vi "Get or Create Virtual Instrument.vi"(8 "Error In":errorcluster, 10 "Virtual Instrument Identifier":string) -> (0 "Error Out":errorcluster, 2 "IVritual Instrument":refnum<class "IVirtual Instrument.lvclass">)   [LabVIEW 2024, in "Instrument Manager.lvclass"]
uses:
  Instrument Manager.lvclass
  Interfaces/IVirtual Instrument/IVirtual Instrument.lvclass
  Instrument Manager.lvclass/Instrument Manager.ctl
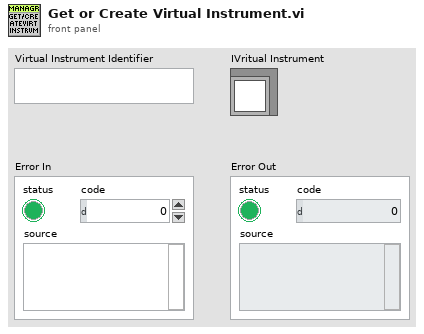
[diagram p1: front panel]
types:
  T1 = map{string, refnum<class "IVirtual Instrument.lvclass">}
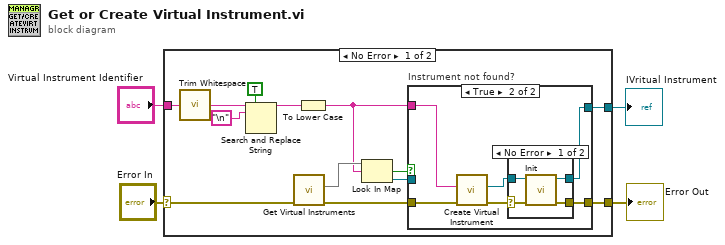
[diagram p0: block diagram]
diagram:
  n1 = case shown="No Error" "Error In" {
    selector: "Error In" -> [w5 w32]
    tunnel: [w17 w32] -> w4
    tunnel: [w12 _] -> w3
    tunnel: "Virtual Instrument Identifier" -> [w11 _]
    frame No Error {
      n2 = call <vilib>:"Trim Whitespace.vi"("string"=w11) -> ("trimmed string"=w7:string)  [unwired: 1 in]
      n3 = Search and Replace String(replace all?=TRUE ("replace all? (F)"), input string=w7, search string="\n") -> (result string=w10:string)  [unwired: 5 in, 3 out]
      n4 = call "Get Virtual Instruments.vi"("Error In"=w5) -> ("Error Out"=w16:errorcluster, "IVirtual Instruments"=w15:T1)  [unwired: 9 in]
      n5 = To Lower Case(string=w10) -> (all lower case string=w6:string)
      n6 = Look In Map(map=w15, key=w6) -> (key not found?=w14:bool, value=w13:refnum<class "IVirtual Instrument.lvclass">)  [unwired: 1 in]
      n7 = case "Instrument not found?" shown="True" w14 {
        tunnel: [w18 w21] -> w17
        tunnel: w16 -> [w18 w24]
        tunnel: w13 -> [w19 _]
        tunnel: [w19 w20] -> w12
        tunnel: w6 -> [_ w23]
        frame False {
        }
        frame True {
          n8 = call "Create Virtual Instrument.vi"("error in"=w24, "Virtual Instrument Identifier"=w23) -> ("error out"=w25:errorcluster, "IVirtual Instrument out"=w22:refnum<class "IVirtual Instrument.lvclass">)  [unwired: 8 in]
          n9 = case shown="No Error" w25 {
            selector: w25 -> [w29 w30]
            tunnel: w22 -> [w28 w31]
            tunnel: [w27 w30] -> w21
            tunnel: [w26 w31] -> w20
            frame No Error {
              n10 = call-dynamic "Init.vi"("error in"=w29, "IInitialize in"=w28) -> ("error out"=w27:errorcluster, "IInitialize out"=w26:refnum<class "IVirtual Instrument.lvclass">)  [unwired: 8 in]
            }
            frame Error {
            }
          }
        }
      }
    }
    frame Error {
    }
  }
  "Error Out" <- w4
  "IVritual Instrument" <- w3
